vi "openImageAndSubBackG.vi"(9 "BG image":T1, 10 "image in":path, 11 "image":T1) -> (2 "BG Out":T1, 3 "raw Image out":T1)   [LabVIEW 2011]
uses:
  IMAQ Image.ctl
  NI_Vision_Development_Module.lvlib
panel:
  out "Boolean":bool
  out "Numeric":i32
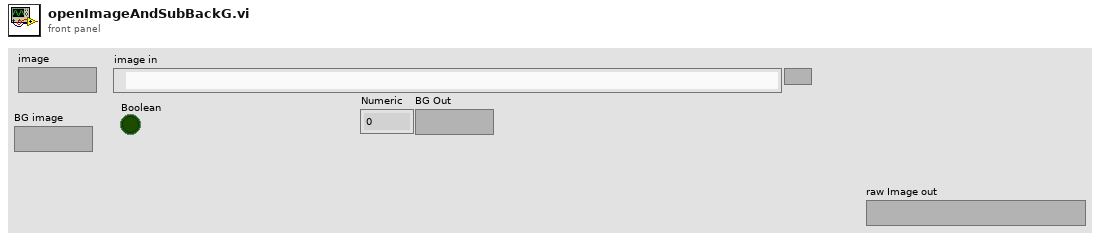
[diagram p1: front panel]
types:
  T1 = typedef "IMAQ Image.ctl" = refnum<image>
  T2 = typedef "Image Type" = u32
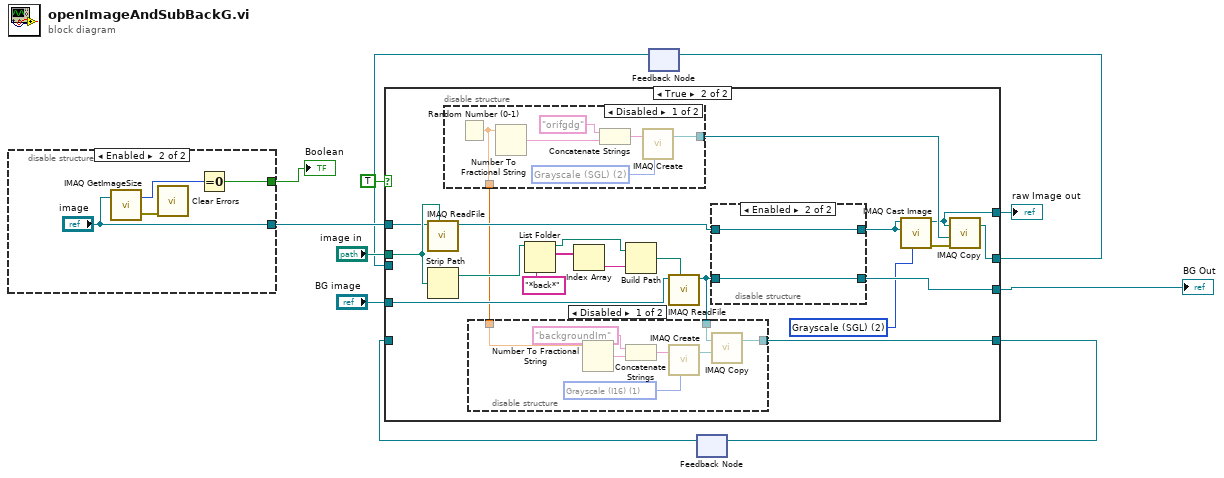
[diagram p0: block diagram]
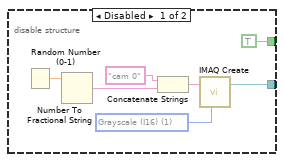
[diagram p2: hidden frame]
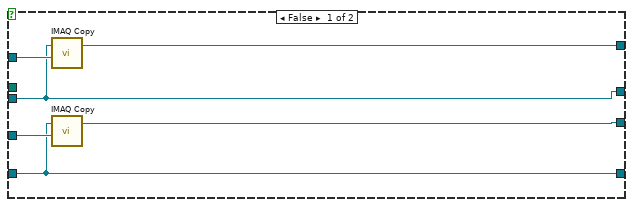
[diagram p3: hidden frame]
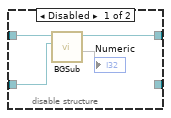
[diagram p6: hidden frame]
diagram:
  n1 = disable-structure shown="Enabled" {
    disable-tunnel: [w13 "image"] -> w10
    disable-tunnel: [TRUE w19] -> w2
    frame Disabled {
      w14 = T2 1 items=["Grayscale (U8)", "Grayscale (I16)", "Grayscale (SGL)", "Complex (CSG)", "RGB (U32)", "HSL (U32)", "RGB (U64)", "Grayscale (U16)"] ("Image Type")
      n2 = Random Number (0-1)() -> (number: 0 to 1=w16:dbl)
      n3 = Number To Fractional String(number=w16) -> (F-format string=w17:string)  [unwired: 3 in]
      n4 = Concatenate Strings("cam 0" ("Image Name"), w17) -> (w18:string)
      n5 = call "IMAQ Create"("Image Name"=w18, "Image Type"=w14) -> ("New Image"=w13:T1)  [unwired: 3 in, 1 out]
    }
    frame Enabled {
      n6 = call "IMAQ GetImageSize"("Image"="image") -> ("Y Resolution"=w22:i32, "error out"=w20:errorcluster)  [unwired: 3 in, 1 out]
      n7 = call "Clear Errors.vi"("error in (no error)"=w20) -> ()  [unwired: 6 in, 1 out]
      n8 = Equal To 0?(x=w22) -> (x = 0?=w19:bool)
    }
  }
  "Boolean" <- w2
  n9 = feedback #1() -> (w6:T1)  [unwired: 1 in]
  n10 = feedback #2() -> (w4:T1)  [unwired: 1 in]
  n11 = case shown="True" TRUE {
    tunnel: [w27 w34] -> w9
    tunnel: "image in" -> [_ w48]
    tunnel: w10 -> [w28 w41]
    tunnel: [w24 w40] -> w8
    tunnel: [w26 w33] -> w7
    tunnel: w6 -> [w26 _]
    tunnel: [w23 w31] -> w5
    tunnel: w4 -> [w23 _]
    tunnel: "BG image" -> [w25 w30]
    frame False {
      n12 = call "IMAQ Copy"("Image Dst"=w28, "Image Src"=w26) -> ("Image Dst Out"=w27:T1)  [unwired: 4 in, 1 out]
      n13 = call "IMAQ Copy"("Image Dst"=w25, "Image Src"=w23) -> ("Image Dst Out"=w24:T1)  [unwired: 4 in, 1 out]
    }
    frame True {
      w38 = T2 2 items=["Grayscale (U8)", "Grayscale (I16)", "Grayscale (SGL)", "Complex (CSG)", "RGB (U32)", "HSL (U32)", "RGB (U64)", "Grayscale (U16)"] ("Image Type")
      n14 = call "IMAQ ReadFile"("File Path"=w48, "Image"=w41) -> ("Image Out"=w36:T1)  [unwired: 5 in, 4 out]
      n15 = Strip Path(path=w48) -> (stripped path=w47:path)  [unwired: 1 out]
      n16 = disable-structure shown="Disabled" {
        disable-tunnel: [w59 _] -> w37
        disable-tunnel: [w57 _] -> w29
        frame Disabled {
          w62 = T2 2 items=["Grayscale (U8)", "Grayscale (I16)", "Grayscale (SGL)", "Complex (CSG)", "RGB (U32)", "HSL (U32)", "RGB (U64)", "Grayscale (U16)"] ("Image Type")
          n17 = Random Number (0-1)() -> (number: 0 to 1=w57:dbl)
          n18 = Number To Fractional String(number=w57) -> (F-format string=w61:string)  [unwired: 3 in]
          n19 = Concatenate Strings("orifgdg" ("Image Name"), w61) -> (w58:string)
          n20 = call "IMAQ Create"("Image Name"=w58, "Image Type"=w62) -> ("New Image"=w59:T1)  [unwired: 3 in, 1 out]
        }
        frame Enabled {
        }
      }
      n21 = List Folder(path=w47, pattern="*back*") -> (path out=w44:path, filenames=w45:string[])  [unwired: 2 in, 2 out]
      n22 = Index Array(array=w45) -> (element=w43:string)  [unwired: 1 in]
      n23 = Build Path(base path=w44, name or relative path=w43) -> (appended path=w42:path)
      n24 = call "IMAQ ReadFile"("File Path"=w42, "Image"=w30) -> ("Image Out"=w32:T1)  [unwired: 5 in, 4 out]
      n25 = disable-structure shown="Disabled" {
        disable-tunnel: w32 -> [w52 _]
        disable-tunnel: [w50 _] -> w31
        disable-tunnel: w29 -> [w49 _]
        frame Disabled {
          w53 = T2 1 items=["Grayscale (U8)", "Grayscale (I16)", "Grayscale (SGL)", "Complex (CSG)", "RGB (U32)", "HSL (U32)", "RGB (U64)", "Grayscale (U16)"] ("Image Type")
          n26 = Number To Fractional String(number=w49) -> (F-format string=w54:string)  [unwired: 3 in]
          n27 = Concatenate Strings("backgroundIm" ("Image Name"), w54) -> (w56:string)
          n28 = call "IMAQ Create"("Image Name"=w56, "Image Type"=w53) -> ("New Image"=w51:T1)  [unwired: 3 in, 1 out]
          n29 = call "IMAQ Copy"("Image Dst"=w51, "Image Src"=w52) -> ("Image Dst Out"=w50:T1)  [unwired: 4 in, 1 out]
        }
        frame Enabled {
        }
      }
      n30 = disable-structure shown="Enabled" {
        disable-tunnel: w36 -> [w66 w68]
        disable-tunnel: w32 -> [w65 w67]
        disable-tunnel: [w64 w68] -> w39
        disable-tunnel: [_ w67] -> w40
        frame Disabled {
          n31 = call "BGSub.vi"("BG IN"=w65, "raw Image In"=w66) -> (1:→"Numeric", "Refnum out"=w64:T1)  [unwired: 6 in, 2 out]
        }
        frame Enabled {
        }
      }
      n32 = call "IMAQ Cast Image"("Image Type"=w38, "Image Dst"=w39, "Image Src"=w39) -> ("error out"=w35:errorcluster, "Image Dst Out"=w34:T1)  [unwired: 7 in]
      n33 = call "IMAQ Copy"("error in (no error)"=w35, "Image Dst"=w37, "Image Src"=w34) -> ("Image Dst Out"=w33:T1)  [unwired: 3 in, 1 out]
    }
  }
  "raw Image out" <- w9
  "BG Out" <- w8
  n34 = feedback-in #1(w7) -> ()
  n35 = feedback-in #2(w5) -> ()
